vi "串口数据处理.vi"(6 "位移输入":dbl[](array[numeric]), 9 "载荷输入":dbl[](array[numeric]), 10 "电量输入":dbl[](array[numeric]), 11 "read buffer":string) -> (1 "当前汇聚节点编号":i32[](array[numeric]), 2 "当前终端节点编号":i32[](array[numeric]), 3 "电量输出":dbl[](array[numeric]), 4 "位移输出":dbl[](array[numeric]), 5 "载荷输出":dbl[](array[numeric]), 7 "当前连接终端节点数量":dbl)   [LabVIEW 2018]
uses:
  <vilib>/regexp/Match Regular Expression.xnode
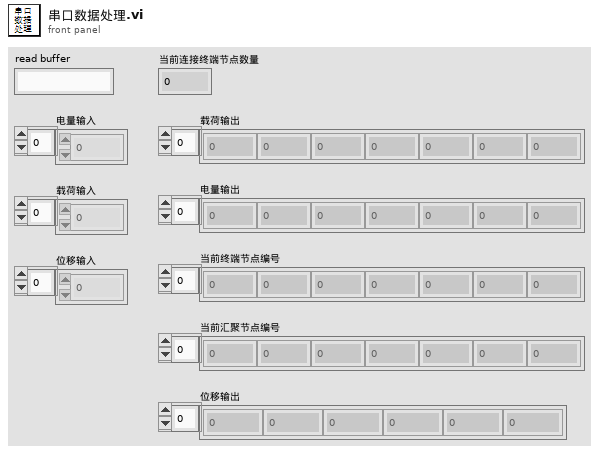
[diagram p1: front panel]
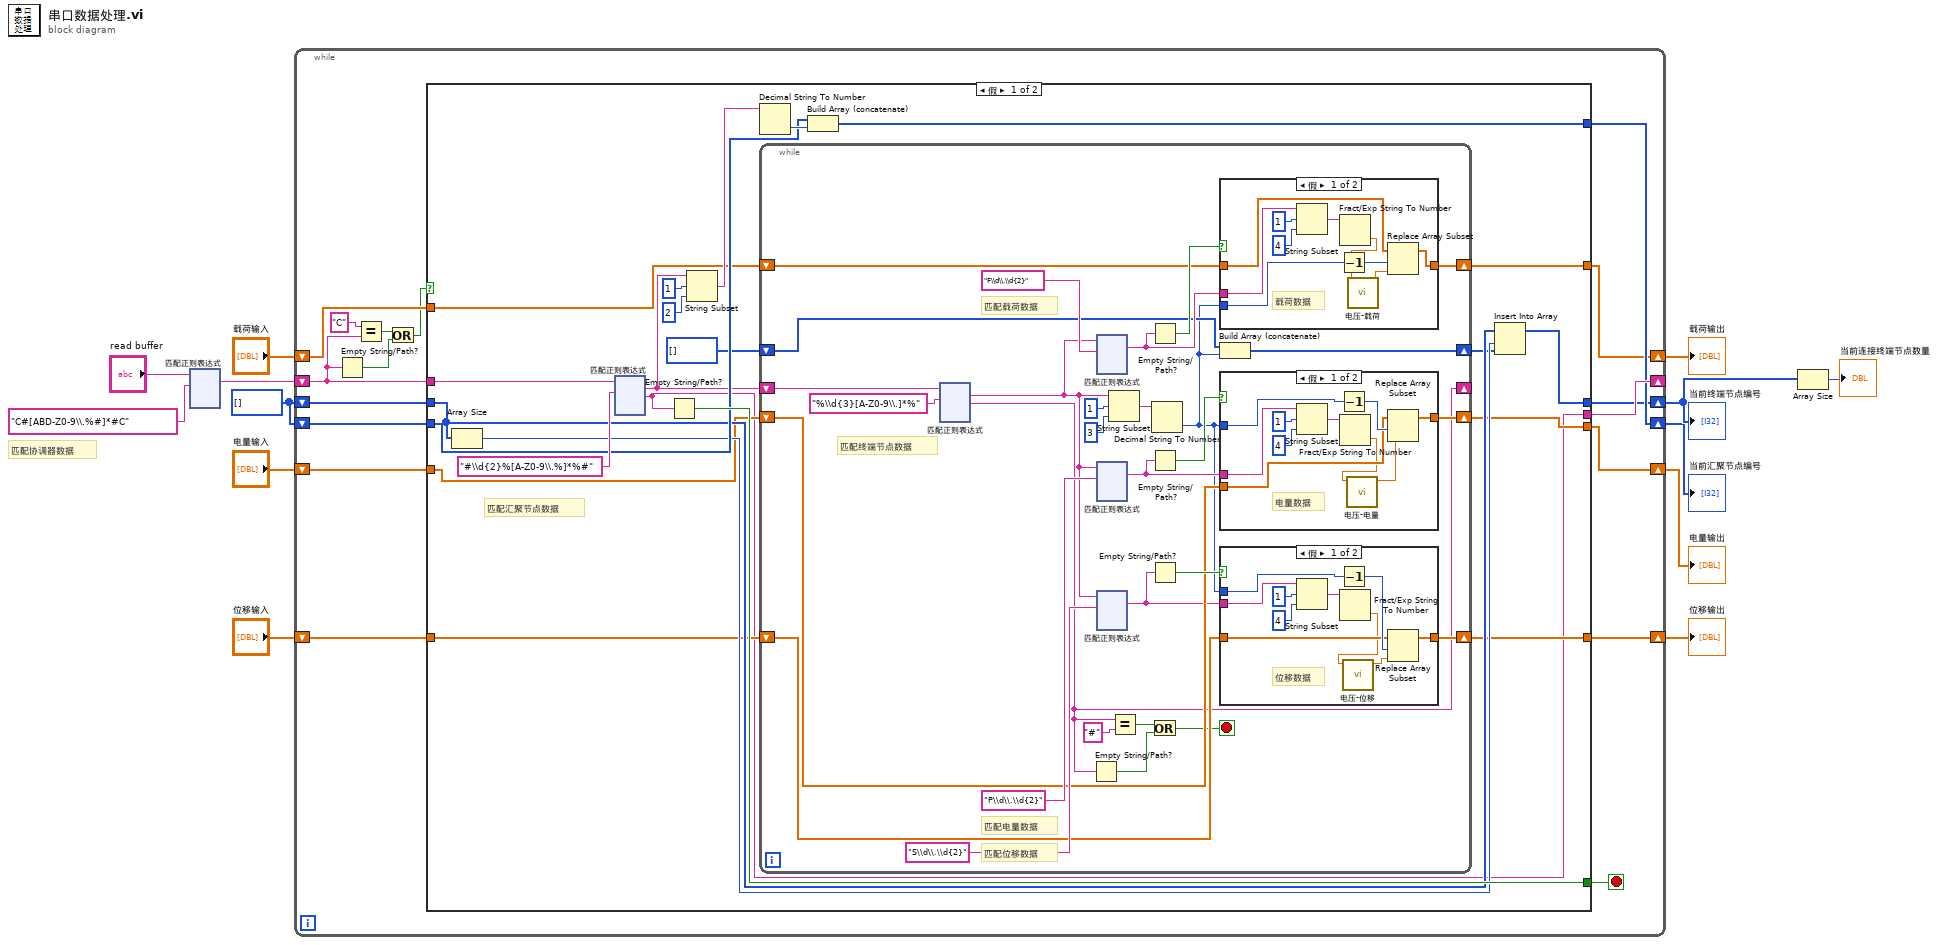
[diagram p0: block diagram]
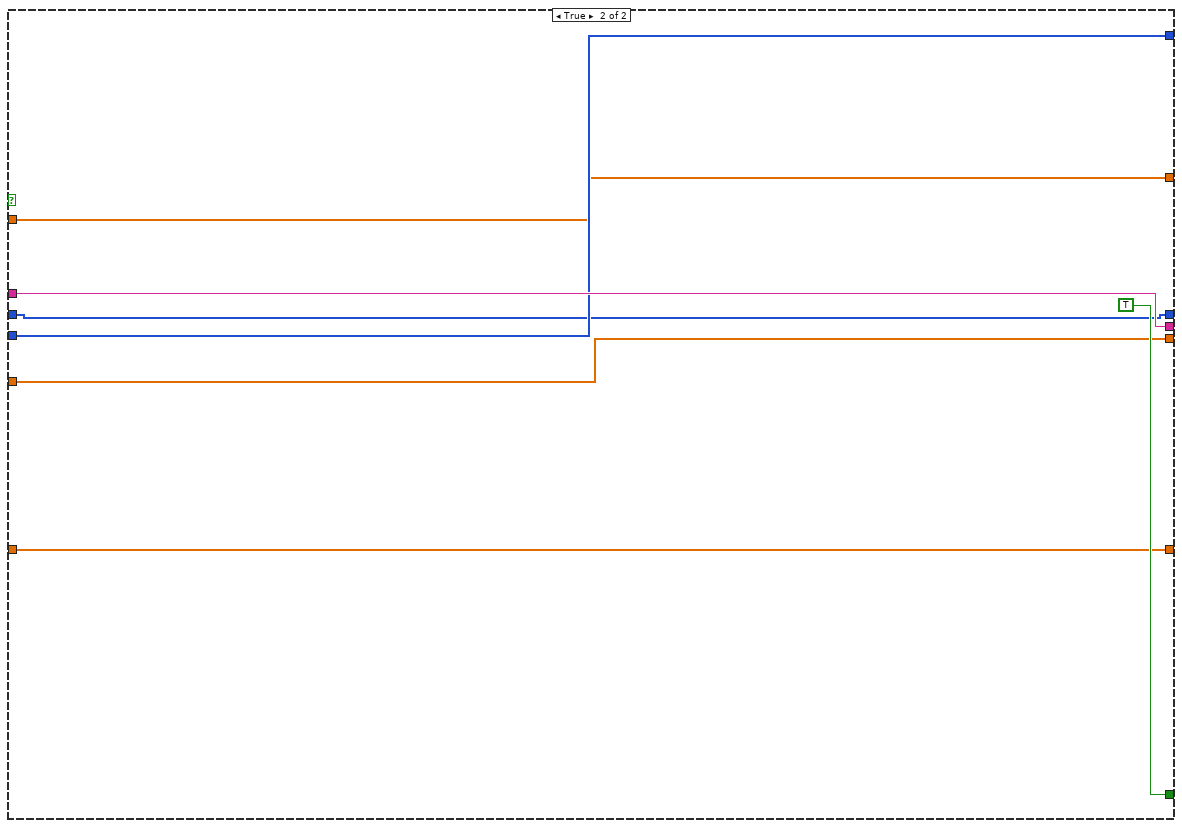
[diagram p5: hidden frame]
diagram:
  w12 = i32[] []
  # "匹配协调器数据"
  n1 = xnode "匹配正则表达式"("输入字符串"="read buffer", "正则表达式"="C#[ABD-Z0-9\\.%#]*#C") -> ("所有匹配"=w6:string)  [unwired: 4 in, 4 out]
  n2 = while {
    shift-right: [w29] -> _
    shift-left: w6 -> [w19]
    shift-right: [w15] -> w2
    shift-left: "载荷输入" -> [w28]
    shift-right: [w26] -> w1
    shift-left: "位移输入" -> [w27]
    shift-right: [w14] -> w3
    shift-left: "电量输入" -> [w25]
    shift-right: [w23] -> w10
    shift-left: w12 -> [w24]
    shift-right: [w21] -> w13
    shift-left: w12 -> [w22]
    stop <- w30 stop-if-true
    n3 = Empty String/Path?(string/path=w19) -> (empty?=w17:bool)
    n4 = Equal?(x="C", y=w19) -> (x = y?=w18:bool)
    n5 = Or(x=w18, y=w17) -> (x .or. y?=w16:bool)
    n6 = case shown="假" w16 {
      tunnel: w19 -> [w52 w691]
      tunnel: [w50 TRUE] -> w30
      tunnel: [w32 w691] -> w29
      tunnel: w28 -> [w38 w686]
      tunnel: [w36 w685] -> w14
      tunnel: w27 -> [w35 w689]
      tunnel: [w34 w689] -> w26
      tunnel: w25 -> [w37 w685]
      tunnel: [w31 w686] -> w15
      tunnel: w24 -> [w45 w688]
      tunnel: [w44 w688] -> w23
      tunnel: w22 -> [w41 w687]
      tunnel: [w39 w687] -> w21
      frame False {
        # "匹配汇聚节点数据"
        n7 = Array Size(array=w41) -> (size(s)=w42:i32)
        n8 = xnode "匹配正则表达式"("输入字符串"=w52, "正则表达式"="#\\d{2}%[A-Z0-9\\.%]*%#") -> ("所有匹配"=w33:string, "匹配之后"=w32:string)  [unwired: 4 in, 3 out]
        n9 = Empty String/Path?(string/path=w32) -> (empty?=w50:bool)
        n10 = String Subset(string=w33, offset (0)=1 ("偏移量(0)"), length (rest)=2 ("长度（剩余）")) -> (substring=w47:string)
        n11 = Decimal String To Number(string=w47) -> (number=w46:i32)  [unwired: 2 in, 1 out]
        n12 = while {
          shift-right: [w53] -> _
          shift-left: w33 -> [w81]
          shift-right: [w68] -> w40
          shift-left: i32[] [] -> [w69]
          shift-right: [w65] -> w31
          shift-left: w38 -> [w66]
          shift-right: [w62] -> w36
          shift-left: w37 -> [w63]
          shift-right: [w58] -> w34
          shift-left: w35 -> [w59]
          stop <- w56 stop-if-true
          # "匹配电量数据"
          # "匹配位移数据"
          # "匹配载荷数据"
          # "匹配终端节点数据"
          n13 = xnode "匹配正则表达式"("输入字符串"=w81, "正则表达式"="%\\d{3}[A-Z0-9\\.]*%") -> ("所有匹配"=w70:string, "匹配之后"=w53:string)  [unwired: 4 in, 3 out]
          n14 = Empty String/Path?(string/path=w53) -> (empty?=w57:bool)
          n15 = xnode "匹配正则表达式"("输入字符串"=w70, "正则表达式"="F\\d\\.\\d{2}") -> ("所有匹配"=w77:string)  [unwired: 4 in, 4 out]
          n16 = xnode "匹配正则表达式"("输入字符串"=w70, "正则表达式"="P\\d\\.\\d{2}") -> ("所有匹配"=w64:string)  [unwired: 4 in, 4 out]
          n17 = xnode "匹配正则表达式"("输入字符串"=w70, "正则表达式"="S\\d\\.\\d{2}") -> ("所有匹配"=w61:string)  [unwired: 4 in, 4 out]
          n18 = String Subset(string=w70, offset (0)=1 ("偏移量(0)"), length (rest)=3 ("长度（剩余）")) -> (substring=w67:string)
          n19 = Equal?(x=w53, y="#") -> (x = y?=w55:bool)
          n20 = Empty String/Path?(string/path=w77) -> (empty?=w78:bool)
          n21 = Empty String/Path?(string/path=w64) -> (empty?=w73:bool)
          n22 = Empty String/Path?(string/path=w61) -> (empty?=w74:bool)
          n23 = Or(x=w55, y=w57) -> (x .or. y?=w56:bool)
          n24 = Decimal String To Number(string=w67) -> (number=w60:i32)  [unwired: 2 in, 1 out]
          n25 = case shown="假" w78 {
            tunnel: w77 -> [w341 _]
            tunnel: w66 -> [w337 w342]
            tunnel: w60 -> [w335 _]
            tunnel: [w334 w342] -> w65
            frame False {
              # "载荷数据"
              n26 = String Subset(string=w341, offset (0)=1 ("偏移量(0)"), length (rest)=4 ("长度（剩余）")) -> (substring=w338:string)
              n27 = Decrement(x=w335) -> (x-1=w336:i32)
              n28 = Fract/Exp String To Number(string=w338) -> (number=w332:dbl)  [unwired: 3 in, 1 out]
              n29 = call "电压-载荷.vi"("输出电压"=w332) -> ("载荷"=w333:dbl)  [unwired: 10 in]
              n30 = Replace Array Subset(array=w337, new element=w333, index=w336) -> (w334:dbl[])
            }
            frame True {
            }
          }
          n31 = Build Array (concatenate)(w69, w60) -> (w68:i32[])
          n32 = case shown="假" w73 {
            tunnel: w64 -> [w87 _]
            tunnel: w60 -> [w86 _]
            tunnel: w63 -> [w85 w92]
            tunnel: [w84 w92] -> w62
            frame False {
              # "电量数据"
              n33 = String Subset(string=w87, offset (0)=1 ("偏移量(0)"), length (rest)=4 ("长度（剩余）")) -> (substring=w89:string)
              n34 = Decrement(x=w86) -> (x-1=w88:i32)
              n35 = Fract/Exp String To Number(string=w89) -> (number=w83:dbl)  [unwired: 3 in, 1 out]
              n36 = call "电压-电量.vi"("输出电压"=w83) -> ("电量"=w82:dbl)  [unwired: 10 in]
              n37 = Replace Array Subset(array=w85, new element=w82, index=w88) -> (w84:dbl[])
            }
            frame True {
            }
          }
          n38 = case shown="假" w74 {
            tunnel: w61 -> [w98 _]
            tunnel: w60 -> [w97 _]
            tunnel: w59 -> [w96 w103]
            tunnel: [w95 w103] -> w58
            frame False {
              # "位移数据"
              n39 = String Subset(string=w98, offset (0)=1 ("偏移量(0)"), length (rest)=4 ("长度（剩余）")) -> (substring=w100:string)
              n40 = Decrement(x=w97) -> (x-1=w99:i32)
              n41 = Fract/Exp String To Number(string=w100) -> (number=w94:dbl)  [unwired: 3 in, 1 out]
              n42 = call "电压-位移.vi"("输出电压"=w94) -> ("位移"=w93:dbl)  [unwired: 10 in]
              n43 = Replace Array Subset(array=w96, new element=w93, index=w99) -> (w95:dbl[])
            }
            frame True {
            }
          }
        }
        n44 = Build Array (concatenate)(w45, w46) -> (w44:i32[])
        n45 = Insert Into Array(array=w41, index=w42, new element=w40) -> (w39:i32[])
      }
      frame True {
      }
    }
  }
  "电量输出" <- w3
  "位移输出" <- w1
  "载荷输出" <- w2
  "当前汇聚节点编号" <- w10
  "当前终端节点编号" <- w13
  n46 = Array Size(array=w13) -> (size(s)=→"当前连接终端节点数量":i32)
